vi "IVI basic control panel.vi"() -> ()   [LabVIEW 2009]
uses:
  Global/GPIB Numbers.vi
panel:
  out "Current Output":dbl
  in  "Read Output":bool
  in  "Set Voltage":bool
  out "Voltage Output":dbl
  in  "Voltage":dbl
  in  "Output On/Off":bool
  in  "VL disabled / enabled":bool
  in  "Voltage Limit":dbl
  in  "Current Limit Behavior":enum16{"REGULATE", "TRIP"}(ring)
  in  "Current Limit":dbl
  in  "Configure Power Supply":bool
  in  "stop":bool
  # "On"
  # "Off"
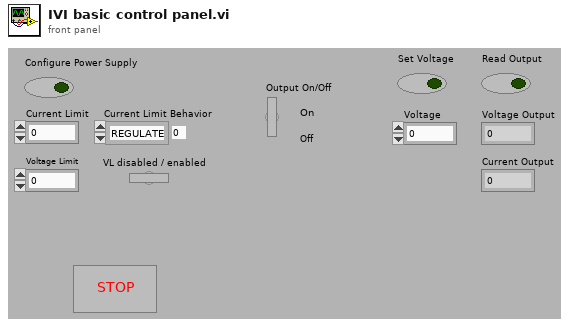
[diagram p1: front panel]
types:
  T1 = cluster{"Name":string, "bus":dbl, "GPIB":dbl, "GPIB as string":string, "byte":i32, "IVI resource name":refnum<k15>, "VISA Resource Name":refnum<visa-resource-name>}
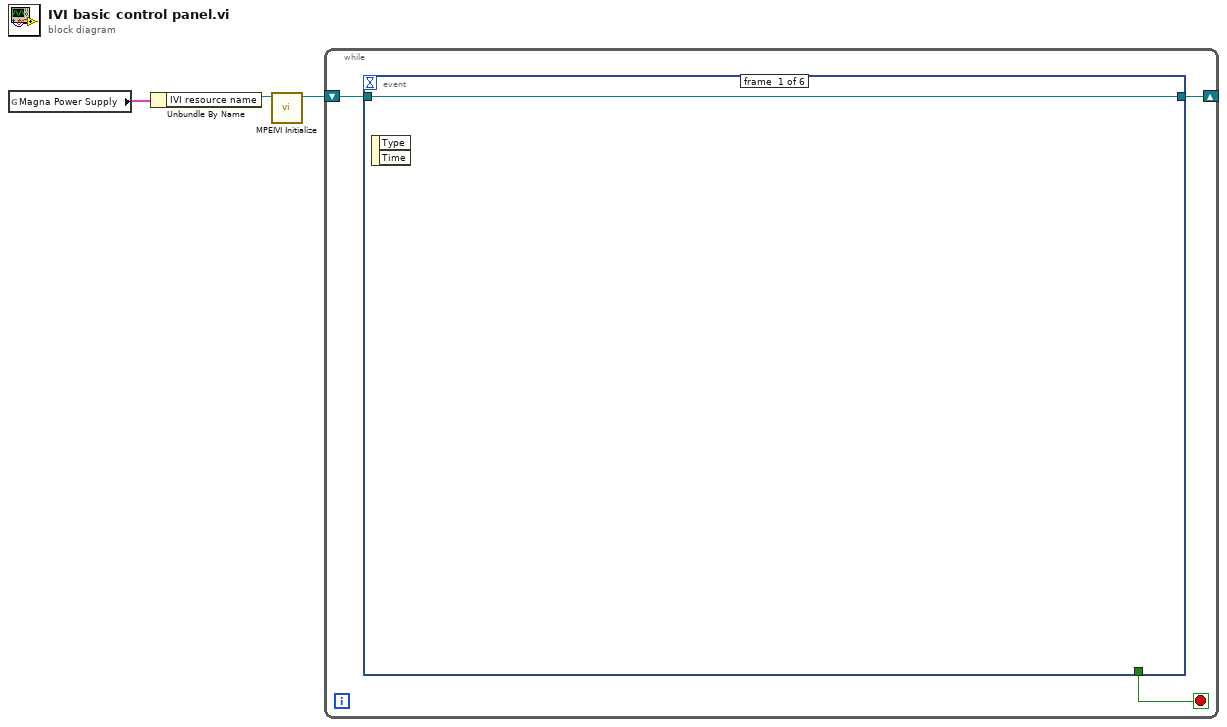
[diagram p0: block diagram]
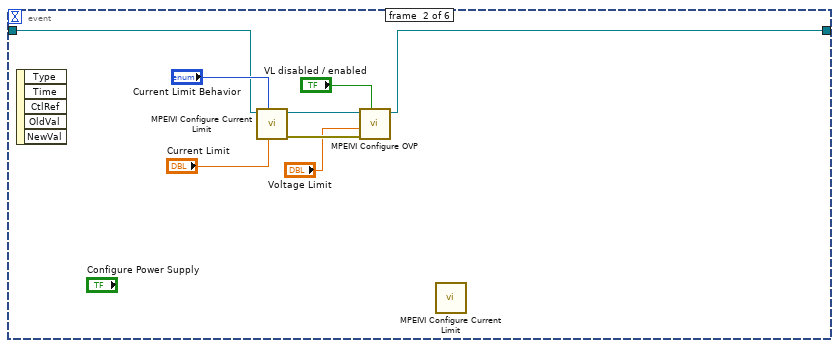
[diagram p2: hidden frame]
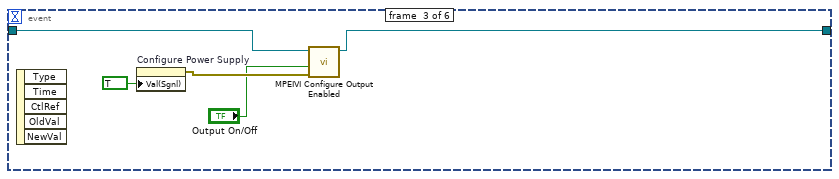
[diagram p3: hidden frame]
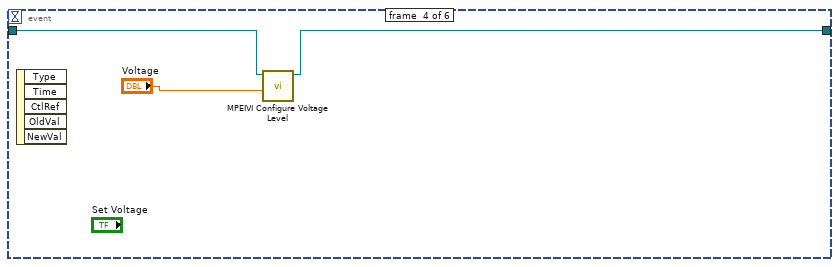
[diagram p4: hidden frame]
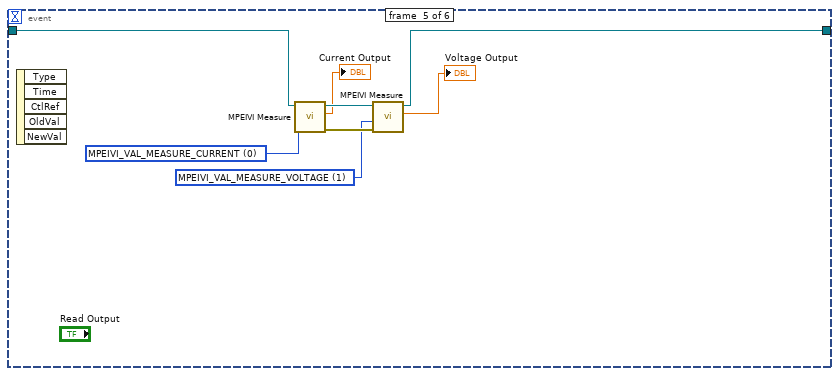
[diagram p5: hidden frame]
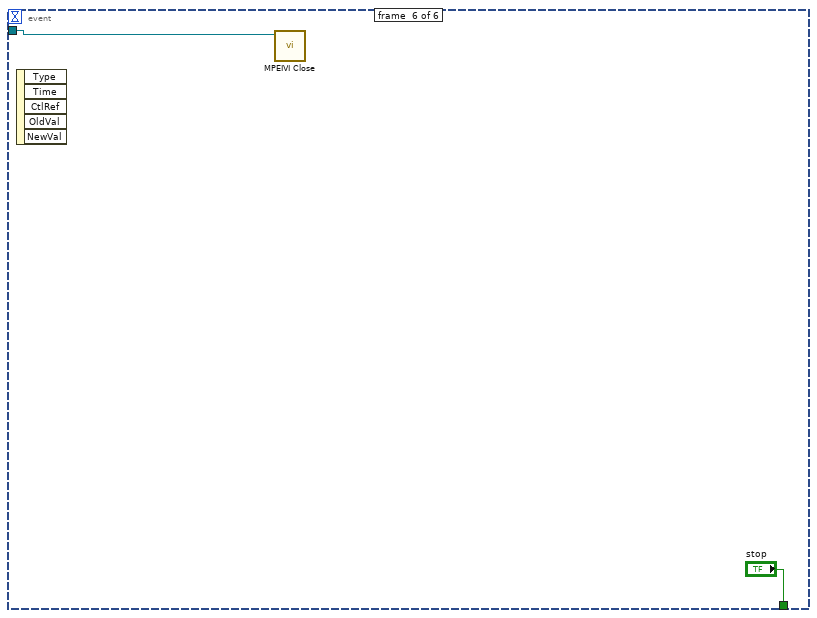
[diagram p6: hidden frame]
diagram:
  n1 = global read "GPIB Numbers.vi" "Magna Power Supply"() -> (w3:T1)
  n2 = Unbundle By Name(w3) -> ("IVI resource name"=w2:refnum<k15>)
  n3 = call <instrlib>:"MPEIVI Initialize.vi"("resource name"=w2) -> ("instrument handle out"=w1:refnum<k15>)  [unwired: 9 in, 1 out]
  n4 = while {
    shift-right: [w4] -> _
    shift-left: w1 -> [w5]
    stop <- w6 stop-if-true
    n5 = event shown="[1] \"Configure Power Supply\": Value Change" {
      selector: _ -> [_ _ _ _ _ _]
      dyn-events: _ -> [_ _ _ _ _ _]
      timeout: _ -> [_ _ _ _ _ _]
      tunnel: [_ _ _ _ _ "stop"] -> w6
      tunnel: w5 -> [w7 w13 w18 w23 w27 w32]
      tunnel: [w7 w8 w16 w21 w24 _] -> w4
      event #0 {
        n6 = event-data() -> ()  [unwired: 1 in, 2 out]
      }
      event #1 {
        n7 = event-data() -> ()  [unwired: 1 in, 5 out]
        n8 = call <instrlib>:"MPEIVI Configure Current Limit.vi"("limit"="Current Limit", "behavior (MPEIVI_VAL_CURRENT_REGULATE)"="Current Limit Behavior", "instrument handle"=w13) -> ("error out"=w11:errorcluster, "instrument handle out"=w12:refnum<k15>)  [unwired: 7 in]
        n9 = call <instrlib>:"MPEIVI Configure OVP.vi"("enabled (Off)"="VL disabled / enabled", "error in (no error)"=w11, "limit"="Voltage Limit", "instrument handle"=w12) -> ("instrument handle out"=w8:refnum<k15>)  [unwired: 6 in, 1 out]
        n10 = call <instrlib>:"MPEIVI Configure Current Limit.vi"() -> ()  [unwired: 10 in, 2 out]
      }
      event #2 {
        n11 = event-data() -> ()  [unwired: 1 in, 5 out]
        n12 = property on="Configure Power Supply" class="Bool (strict)"("Val(Sgnl)"=TRUE ("Value (Signaling)")) -> (error out=w19:errorcluster)  [unwired: 2 in, 1 out]
        n13 = call <instrlib>:"MPEIVI Configure Output Enabled.vi"("error in (no error)"=w19, "enabled (Off)"="Output On/Off", "instrument handle"=w18) -> ("instrument handle out"=w16:refnum<k15>)  [unwired: 7 in, 1 out]
      }
      event #3 {
        n14 = event-data() -> ()  [unwired: 1 in, 5 out]
        n15 = call <instrlib>:"MPEIVI Configure Voltage Level.vi"("level"="Voltage", "instrument handle"=w23) -> ("instrument handle out"=w21:refnum<k15>)  [unwired: 8 in, 1 out]
      }
      event #4 {
        w28 = 1 items=["MPEIVI_VAL_MEASURE_CURRENT", "MPEIVI_VAL_MEASURE_VOLTAGE"] ("measurement type (MPEIVI_VAL_MEASURE_CURRENT)")
        w31 = 0 items=["MPEIVI_VAL_MEASURE_CURRENT", "MPEIVI_VAL_MEASURE_VOLTAGE"] ("measurement type (MPEIVI_VAL_MEASURE_CURRENT)")
        n16 = event-data() -> ()  [unwired: 1 in, 5 out]
        n17 = call <instrlib>:"MPEIVI Measure.vi"("measurement type (MPEIVI_VAL_MEASURE_CURRENT)"=w31, "instrument handle"=w27) -> ("error out"=w29:errorcluster, "measurement"=→"Current Output":dbl, "instrument handle out"=w30:refnum<k15>)  [unwired: 7 in]
        n18 = call <instrlib>:"MPEIVI Measure.vi"("error in (no error)"=w29, "measurement type (MPEIVI_VAL_MEASURE_CURRENT)"=w28, "instrument handle"=w30) -> ("measurement"=→"Voltage Output":dbl, "instrument handle out"=w24:refnum<k15>)  [unwired: 6 in, 1 out]
      }
      event #5 {
        n19 = event-data() -> ()  [unwired: 1 in, 5 out]
        n20 = call <instrlib>:"MPEIVI Close.vi"("instrument handle"=w32) -> ()  [unwired: 10 in, 1 out]
      }
    }
  }
